vi "Pad Boolean Array.vi"(1 "Boolean array in":bool[](array[boolean])) -> (0 "Padded array":bool[](array[boolean]))   [LabVIEW 2021, in "FPGA Register IO Tests.lvclass"]
uses:
  FPGA Register IO Tests.lvclass
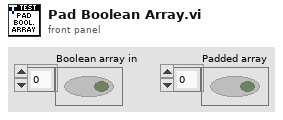
[diagram p1: front panel]
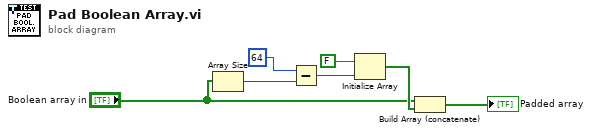
[diagram p0: block diagram]
diagram:
  n1 = Array Size(array="Boolean array in") -> (size(s)=w2:i32)
  n2 = Subtract(x=64, y=w2) -> (x-y=w3:i32)
  n3 = Initialize Array(FALSE, w3) -> (w6:bool[])
  n4 = Build Array (concatenate)("Boolean array in", w6) -> (→"Padded array":bool[])
